vi "SEA_POSITION_CONTROL.vi"() -> ()   [LabVIEW 2019]
uses:
  <vilib>/Platform/TimedLoop/XDataNode/timing_clust.ctl
  <vilib>/Platform/TimedLoop/XDataNode/nitl_modes.ctl
  <vilib>/Platform/TimedLoop/XDataNode/wakeup.ctl
  <vilib>/FPGAPlugInAG/sbRIO-9627/niLvFpga_Open_sbRIO-9627.vi
  <vilib>/rvi/interface/common/dynamic/niFpgaDynamicAddResources.vi
  <vilib>/Utility/error.llb/Error Cluster From Error Code.vi
  <vilib>/rvi/errors/niLvFpgaAdjustHostInterfaceError.vi
  <vilib>/FPGAPlugInAG/Dynamic/niLvFpga_Close_Dynamic.vi
  <vilib>/rvi/interface/nirviOpenFPGA/nirviOpenFPGA.xnode
  FPGA Bitfiles/seafinalexperime_FPGATarget_SEALOWERLEVELCON_meT+vsors+U.lvbitx
  SEA_LOWER_LEVEL_CONTROL.vi
  <vilib>/platform/TimedLoop/XDataNode/XDataNode.xnode
  <vilib>/rvi/interface/nirviReadWriteControl/nirviReadWriteControl.xnode
  <vilib>/rvi/interface/nirviCloseFPGA/nirviCloseFPGA.xnode
  NiFpgaLv.dll
  <vilib>/rvi/interface/Simulation/niFpgaSimulationCallBeginRW.vi
  <vilib>/Platform/TimedLoop/XDataNode/XDNodeRunTimeDep.lvlib
panel:
  out "Finished late count":u32
  in  "lower limit":sgl
  in  "upper limit":sgl
  in  "Kp":sgl
  in  "KpGain":sgl
  out "Motor current":T1(graph)
  out "Joint position":cluster{sgl, "Position(Radians) joint side":sgl}(graph)
  in  "stop":bool
  in  "Tracking zero offset":sgl
  in  "Current Offset":sgl
  in  "Amplitude":sgl
  in  "frequency":sgl
  in  "Position Reset":bool
  in  "Position Reset joint side":bool
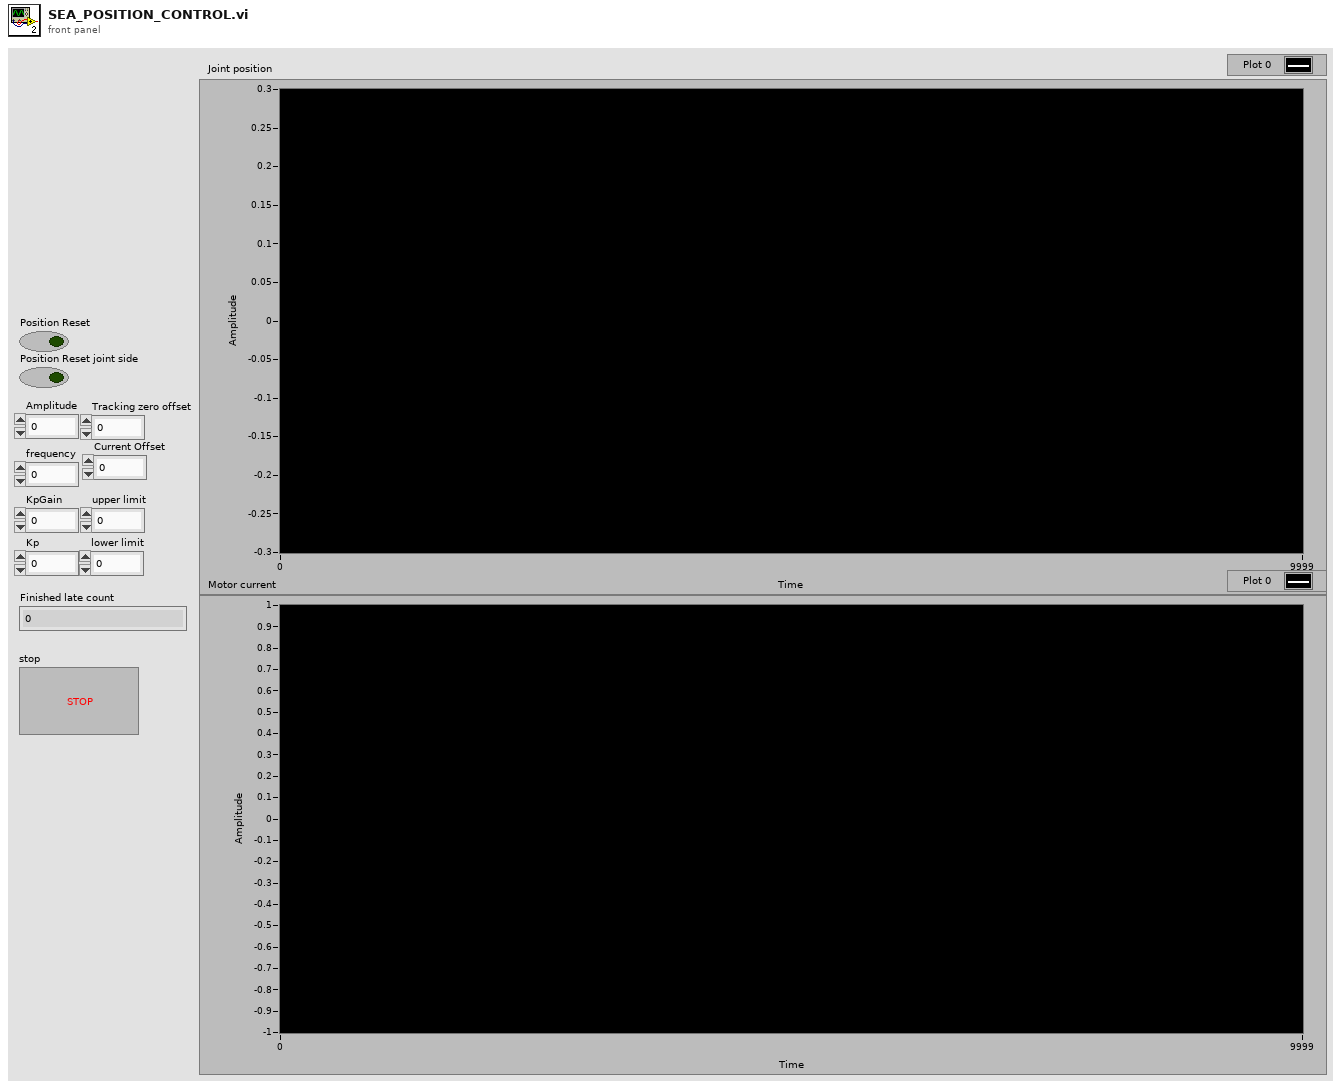
[diagram p1: front panel]
types:
  T1 = cluster{"upper limit":sgl, "Filtered Current(M2)":sgl}
  T2 = typedef "XDNodeRunTimeDep.lvlib/timing_clust.ctl" = cluster{"Expected End [f-1]":u64, "Actual End [f-1]":u64, "Finished Late? [f-1]":bool, "Expected End [i-1]":u64, "Actual End [i-1]":u64, "Finished Late? [i-1]":bool, "Expected Start [i]":u64, "Actual Start [i]":u64, "Expected Start [f]":u64, "Actual Start [f]":u64, "Source Name":string, "Structure Name":string, "Period":i64, "Deadline":i64, "Offset":i64, "Start":i64, "Priority":i32, "Timeout":i32, "Mode":T3, "Wakeup Reason":T4, "Error":errorcluster, "Source Type":string, "Secondary Source Type":string, "Global End Time":u64, "Global Start Time":u64, "Frame Duration":u64, "Iteration Duration":u64, "Assigned CPU":i32, "I/O Scan Engine Mode":u32}
  T3 = typedef "XDNodeRunTimeDep.lvlib/nitl_modes.ctl" = enum32{"No Change", "Process missed periods, maintain original phase", "Discard missed periods, maintain original phase", "Process missed periods, ignore original phase", "Discard missed periods, ignore original phase"}
  T4 = typedef "XDNodeRunTimeDep.lvlib/wakeup.ctl" = enum32{"Normal", "Aborted", "Asynchronous wakeup", "Timing source error", "Timed loop error", "Timeout"}
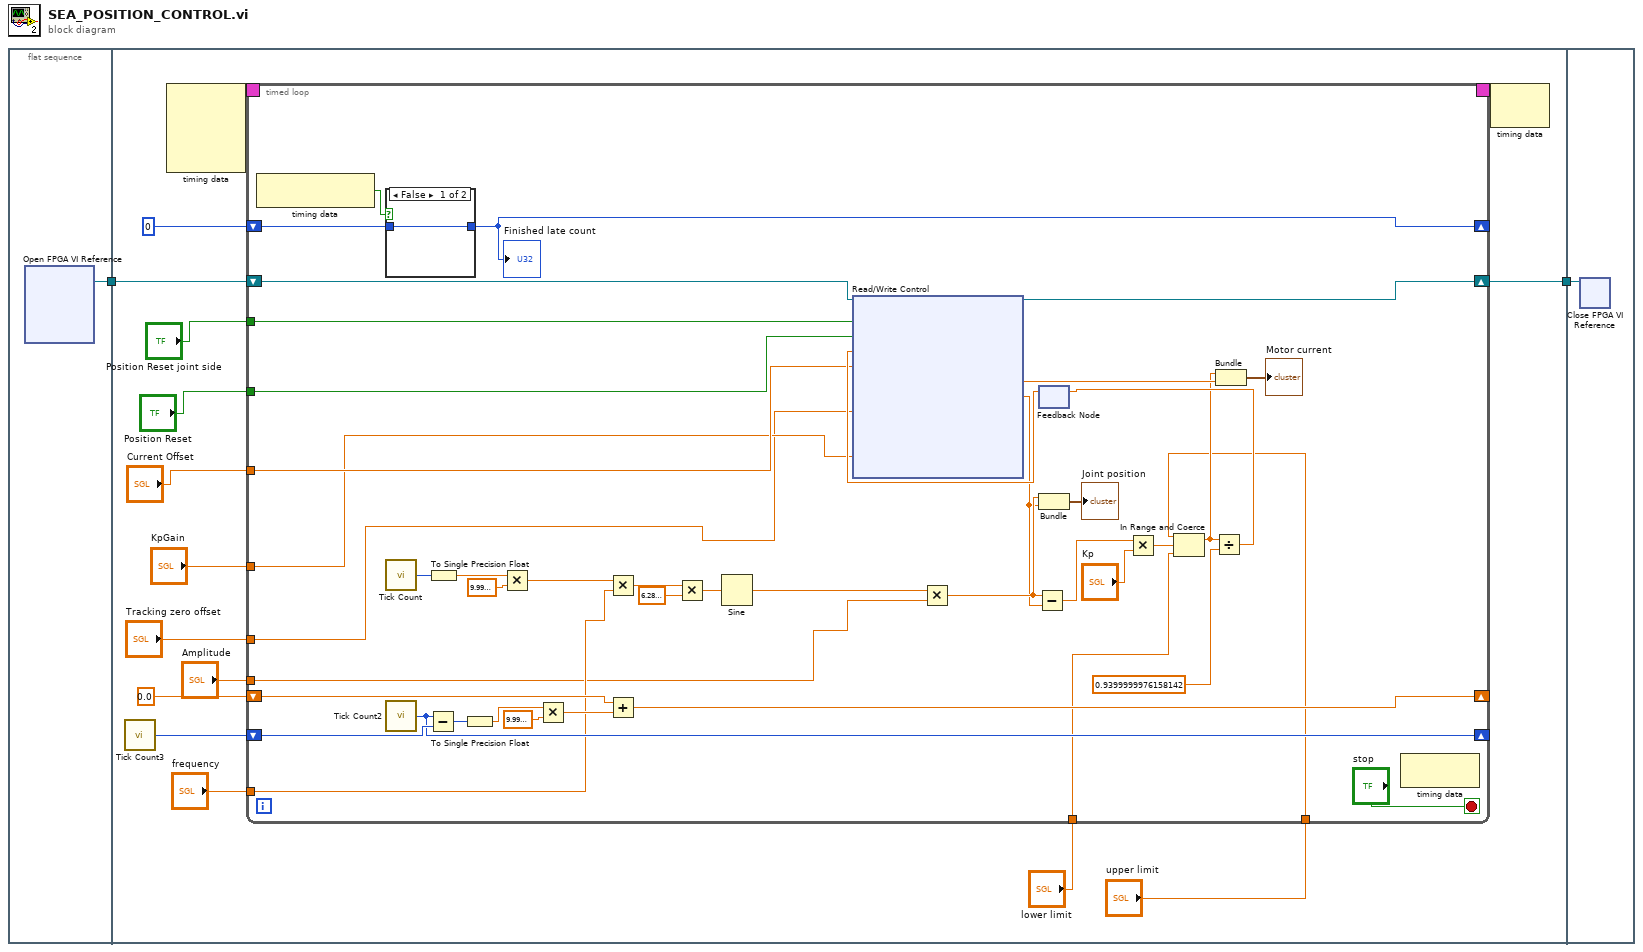
[diagram p0: block diagram]
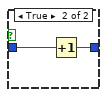
[diagram p2: hidden frame]
diagram:
  n1 = flat-sequence {
    tunnel: [w3] -> w2
    tunnel: w2 -> [w19]
    tunnel: [w18] -> w1
    tunnel: w1 -> [w71]
    frame #0 {
      n2 = xnode "Open FPGA VI Reference"() -> ("FPGA VI Reference Out"=w3:refnum<k20>)  [unwired: 2 in, 1 out]
    }
    frame #1 {
      n3 = call "Tick Count3"() -> ("Tick Count(uSec)"=w17:u32)
      n4 = node-c288() -> (w15:T2)  [unwired: 4 in]
      n5 = timed-loop {
        shift-right: [w44] -> w18
        shift-left: w19 -> [w62]
        shift-right: [w54] -> _
        shift-left: w17 -> [w58]
        shift-right: [w51] -> _
        shift-left: sgl 0.0 -> [w52]
        timing: w15 -> [_]
        timing-out: [_] -> w14
        shift-right: [w30] -> _
        shift-left: u32 0 -> [w31]
        tunnel: "Position Reset joint side" -> [w29]
        tunnel: "Position Reset" -> [w28]
        tunnel: "Current Offset" -> [w27]
        tunnel: "KpGain" -> [w26]
        tunnel: "Tracking zero offset" -> [w25]
        tunnel: "frequency" -> [w24]
        tunnel: "Amplitude" -> [w22]
        tunnel: "lower limit" -> [w21]
        tunnel: "upper limit" -> [w20]
        stop <- "stop" stop-if-true
        n6 = node-c288() -> (w32:bool)  [unwired: 1 in]
        n7 = case shown="False" w32 {
          tunnel: w31 -> [w63 w65]
          tunnel: [w63 w64] -> w30
          frame False {
          }
          frame True {
            n8 = Increment(x=w65) -> (x+1=w64:u32)
          }
        }
        "Finished late count" <- w30
        n9 = call "Tick Count"() -> ("Tick Count(uSec)"=w42:u32)
        n10 = call "Tick Count2"() -> ("Tick Count(uSec)"=w54:u32)
        n11 = Subtract(x=w54, y=w58) -> (x-y=w57:u32)
        n12 = To Single Precision Float(number=w42) -> (single precision float=w43:sgl)
        n13 = To Single Precision Float(number=w57) -> (single precision float=w56:sgl)
        n14 = Multiply(x=w43, y=sgl 1e-06) -> (x*y=w40:sgl)
        n15 = Multiply(x=w56, y=sgl 1e-06) -> (x*y=w53:sgl)
        n16 = Multiply(x=w40, y=w24) -> (x*y=w61:sgl)
        n17 = Add(x=w52, y=w53) -> (x+y=w51:sgl)
        n18 = Multiply(x=w61, y=sgl 6.28) -> (x*y=w60:sgl)
        n19 = Sine(x=w60) -> (sin(x)=w50:sgl)
        n20 = Multiply(x=w50, y=w22) -> (x*y=w39:sgl)
        n21 = feedback #1() -> (w46:sgl)  [unwired: 1 in]
        n22 = xnode "Read/Write Control"("FPGA VI Reference In"=w62, "Position Reset joint side"=w29, "Position Reset"=w28, "reference"=w46, "Current Offset"=w27, "Tracking zero offset"=w25, "KpGain"=w26) -> ("FPGA VI Reference Out"=w44:refnum<k20>, "Filtered Current(M2)"=w45:sgl, "Position(Radians) joint side"=w38:sgl)  [unwired: 1 in, 4 out]
        n23 = Subtract(x=w39, y=w38) -> (x-y=w37:sgl)
        n24 = Bundle(w39, "Position(Radians) joint side"=w38) -> (→"Joint position":cluster{sgl, "Position(Radians) joint side":sgl})  [unwired: 1 in]
        n25 = Multiply(x=w37, y="Kp") -> (x*y=w35:sgl)
        n26 = In Range and Coerce(upper limit=w20, x=w35, lower limit=w21) -> (coerced(x)=w34:sgl)  [unwired: 1 out]
        n27 = Divide(x=w34, y=sgl 0.94) -> (x/y=w48:sgl)
        n28 = feedback-in #1(w48) -> ()
        n29 = Bundle("upper limit"=w34, "Filtered Current(M2)"=w45) -> (→"Motor current":T1)  [unwired: 1 in]
        n30 = node-c288() -> ()  [unwired: 1 in, 1 out]
      }
      n31 = node-c288(w14) -> ()  [unwired: 1 out]
    }
    frame #2 {
      n32 = xnode "Close FPGA VI Reference"("FPGA VI Reference In"=w71) -> ()  [unwired: 1 in, 1 out]
    }
  }
